vi "写入表格.vi"(8 "error in (no error)":errorcluster, 9 "section":string="报告表格", 10 "Controls[]":refnum<vi>[](array[refnum]), 11 "引用句柄输入":T1 caption="refnum") -> (0 "错误输出":errorcluster caption="error out", 3 "引用句柄输出":T1 caption="refnum out")   [LabVIEW 2013]
doc: "手动向表格中输入数据，并保存到对应的配置文件里"
uses:
  <vilib>/Utility/config.llb/Config Data RefNum.ctl
  <vilib>/Utility/config.llb/Write Key (String).vi
  <vilib>/Utility/config.llb/NI_LVConfig.lvlib
panel:
  out "Array":bool[](array[boolean])
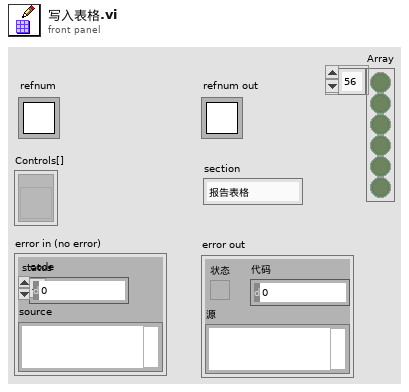
[diagram p1: front panel]
types:
  T1 = typedef "NI_LVConfig.lvlib/Config Data RefNum.ctl" = refnum<k1>
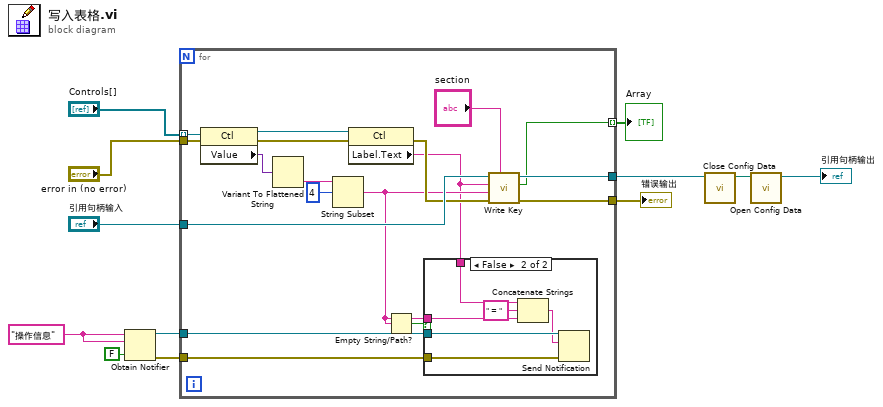
[diagram p0: block diagram]
diagram:
  w8 = "操作信息"
  n1 = Obtain Notifier(name (unnamed)=w8, notification data type=w8, create if not found? (T)=FALSE) -> (notifier out=w7:refnum<notifier>, error out=w6:errorcluster)  [unwired: 1 in, 1 out]
  n2 = for {
    tunnel: "Controls[]" -> [w30] mode=indexing
    tunnel: "引用句柄输入" -> [w27]
    tunnel: [w26] -> w2
    tunnel: [w21] -> w12
    tunnel: w7 -> [w20]
    tunnel: w6 -> [w19]
    tunnel: "error in (no error)" -> [w17]
    tunnel: [w13] -> w4 mode=indexing
    n3 = property class="Ctl"(reference=w30, error in=w17) -> (reference out=w29:refnum<vi>, error out=w23:errorcluster, "Value"=w28:variant)
    n4 = Variant To Flattened String(Variant=w28) -> (data string=w18:string)  [unwired: 1 out]
    n5 = String Subset(string=w18, offset (0)=4 ("偏移量(0)")) -> (substring=w15:string)  [unwired: 1 in]
    n6 = property class="Ctl"(reference=w29, error in=w23) -> (error out=w22:errorcluster, "Label.Text"=w14:string)  [unwired: 1 out]
    n7 = Empty String/Path?(string/path=w15) -> (empty?=w16:bool)
    n8 = case shown="False" w16 {
      tunnel: w20 -> [_ w36]
      tunnel: w19 -> [_ w35]
      tunnel: w15 -> [_ w33]
      tunnel: w14 -> [_ w32]
      frame True {
      }
      frame False {
        n9 = Concatenate Strings(w32, " = " ("string"), w33) -> (w34:string)
        n10 = Send Notification(notification=w34, notifier=w36, error in (no error)=w35) -> ()  [unwired: 2 out]
      }
    }
    n11 = call-poly <vilib>:"Write Key.vi"("section"="section", "error in (no error)"=w22, "value"=w15, "key"=w14, "refnum"=w27) -> ("error out"=w21:errorcluster, "found?"=w13:bool, "refnum out"=w26:T1)  [unwired: 4 in]
  }
  "错误输出" <- w12
  "Array" <- w4
  n12 = call <vilib>:"Close Config Data.vi"("refnum"=w2) -> ("file path"=w3:path)  [unwired: 9 in, 1 out]
  n13 = call <vilib>:"Open Config Data.vi"("configuration file path"=w3) -> ("refnum"=→"引用句柄输出":T1)  [unwired: 8 in, 2 out]
